vi "QueryServer_GetRequest_Register.vi"(0 "gRPCid":T1, 3 "error in (no error)":errorcluster) -> (7 "gRPCid out":T1, 9 "eventname":string, 10 "error out":errorcluster)   [LabVIEW 2019, in "labview-grpc-query-server.lvlib"]
uses:
  labview-grpc-query-server.lvlib
  gRPC interface/Server API/typeDefs/grpcId.ctl
  QueryServer_RegisterRequest.ctl
  70238de4-b0bb-4b1d-82fe-e867cd1b1217.vi
  gRPC interface/gprc-lvsupport.lvlib
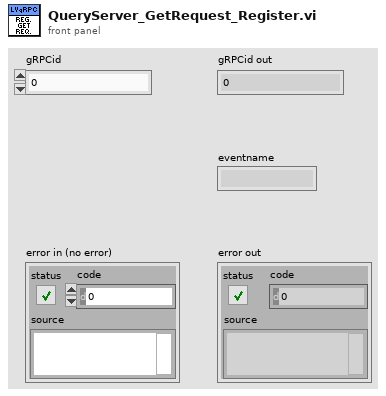
[diagram p1: front panel]
types:
  T1 = typedef "gprc-lvsupport.lvlib/grpcId.ctl" = u64
  T2 = typedef "labview-grpc-query-server.lvlib/QueryServer_RegisterRequest.ctl" = cluster{"eventname":string}
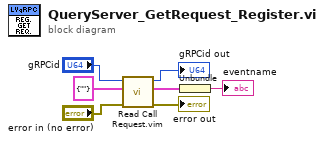
[diagram p0: block diagram]
diagram:
  n1 = call "Read Call Request.vim"("error in (no error)"="error in (no error)", "Data Type"=T2 {"eventname"=""} ("RegistrationRequest"), "gRPCid in"="gRPCid") -> ("error out"=→"error out":errorcluster, "Request Data"=w6:T2, "gRPCid out"=→"gRPCid out":T1)  [unwired: 6 in]
  n2 = Unbundle(w6) -> ("eventname"=→"eventname":string)
